vi "stream.create.vi"(7 "fallback avro file (user documents\\nominal_fallback_files)":path, 8 "error in (no error)":errorcluster, 11 "dataset in":refnum<class "dataset.lvclass">) -> (0 "error out":errorcluster, 2 "Stream":refnum<class "Stream.lvclass">, 3 "dataset out":refnum<class "dataset.lvclass">)   [LabVIEW 2020, in "datasources.lvlib" / "dataset.lvclass"]
uses:
  dataset.lvclass
  submodules/nominal-streaming-labview-ffi/lv_src/Stream/Stream.lvclass
  <vilib>/Utility/sysdir.llb/System Directory Type.ctl
  dataset.lvclass/dataset.ctl
  Nominal Client/Nominal Client.lvclass/Nominal Client.ctl
  Nominal Client/Nominal Client.lvclass
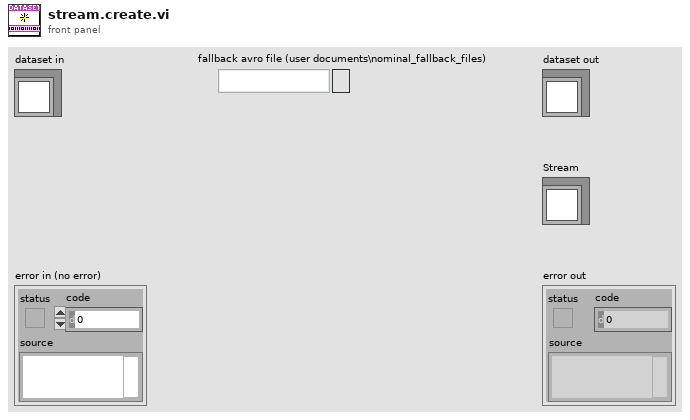
[diagram p1: front panel]
types:
  T1 = typedef "System Directory Type.ctl" = i32
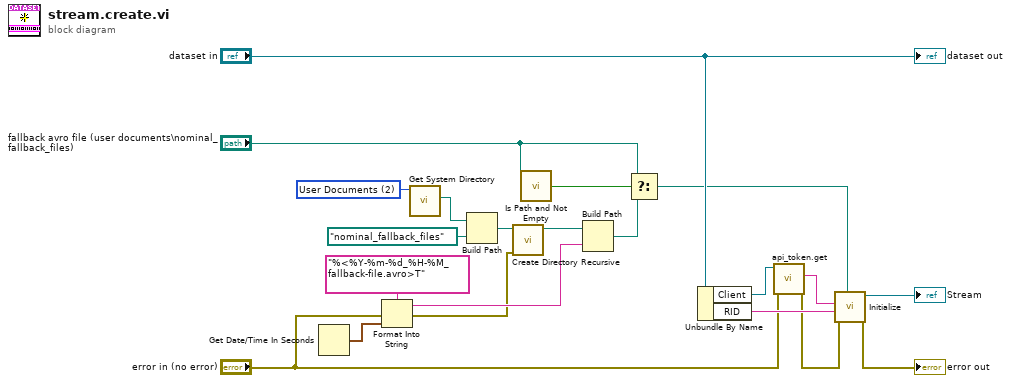
[diagram p0: block diagram]
diagram:
  w12 = T1 2 items=["User Home"=0, "User Desktop"=1, "User Documents"=2, "User Application Data"=3, "User Preferences"=4, "User Temporary"=5, "Public Documents"=6, "Public Application Data"=7, "Public Preferences"=8, "Public Cache"=13, "System Core Libraries"=9, "System Installed Libraries"=10, "Application Files"=11, "Boot Volume Root"=12] ("system directory type")
  n1 = Get Date/Time In Seconds() -> (seconds since 1Jan1904=w15:timestamp)
  n2 = Format Into String(format string="%<%Y-%m-%d_%H-%M_fallback-file.avro>T", error in="error in (no error)", w15) -> (resulting string=w14:string, error out=w9:errorcluster)  [unwired: 1 in]
  n3 = call <vilib>:"Get System Directory.vi"("system directory type"=w12) -> ("system directory"=w13:path)  [unwired: 10 in]
  n4 = Build Path(base path=w13, name or relative path=path "nominal_fallback_files") -> (appended path=w11:path)
  n5 = call <vilib>:"Create Directory Recursive.vi"("error in (no error)"=w9, "directory"=w11) -> ("directory copy"=w10:path)  [unwired: 3 in, 2 out]
  n6 = call <vilib>:"Is Path and Not Empty.vi"("path"="fallback avro file (user documents\\nominal_fallback_files)") -> ("Is Path and Not Empty?"=w8:bool)  [unwired: 4 in]
  n7 = Build Path(base path=w10, name or relative path=w14) -> (appended path=w6:path)
  n8 = Select(t="fallback avro file (user documents\\nominal_fallback_files)", s=w8, f=w6) -> (s? t:f=w5:path)
  n9 = Unbundle By Name("dataset in") -> ("Client"=w3:refnum<class "Nominal Client.lvclass">, "RID"=w18:string)
  n10 = call "api_token.get.vi"("error in"="error in (no error)", "Nominal Client in"=w3) -> ("error out"=w1:errorcluster, "API Token"=w4:string)  [unwired: 7 in, 1 out]
  n11 = call "Initialize.vi"("Fallback File Path"=w5, "error in (no error)"=w1, "Dataset RID"=w18, "Token"=w4) -> ("error out"=→"error out":errorcluster, "Nominal Streaming out"=→"Stream":refnum<class "Stream.lvclass">)  [unwired: 6 in]
  "dataset out" <- "dataset in"
